vi "Serial Write and Read.vi"() -> ()   [LabVIEW 2019]
doc: "This example performs writes and reads on a serial port, as directed by the user. You can press the Write and Read buttons, and change the Read Count, while the example is running.\n\nThe parameters set for the serial port must match the parameters of the connected instrument or device. In this example, the Read Count parameter specifies the number of bytes that the serial port reads. If there were more bytes at the port than the specified number, those bytes would not be read. If there were less bytes at the port than the specified number, you would receive a timeout error.\n\nThis example expands upon the flow control options for XON and XOFF, allowing the user to choose those control characters. Also, the user can enable or disable a termination character. Some devices require a termination character in order to identify the end of command strings. Some devices send a termination character to signify the end of data to be read. This example shows how you can end the Read operation once a termination character is detected in the buffer and/or append a termination character at the end of the Write data."
uses:
  C:/Program Files (x86)/National Instruments/LabVIEW 2019/examples/Instrument IO/Serial/support/Serial - Settings.ctl
  <vilib>/Math Plots/3D Math Plots/3D Surface/3D Surface XCtrl/3D Surface.xctl
  <vilib>/Instr/_visa.llb/VISA Configure Serial Port (Instr).vi
  <vilib>/Math Plots/3D Math Plots/3D Surface/3D Surface Datatype/Public/Plot Helper (Vector).vi
  <vilib>/Utility/file.llb/Write Delimited Spreadsheet (string).vi
  <vilib>/Analysis/NI_AALBase.lvlib
  <vilib>/Math Plots/3D Math Plots/3D Surface/3D Surface Datatype/3D Surface Datatype.lvclass
panel:
  out "Noisy Pixel List":i32[][](array[numeric])
  out "Elapsed Time":dbl format="%#_g s"
  out "Intensity Graph":u32[][](graph)
  out "Cleaned Data":string[](array[string])
  out "Numeric Control":i32
  out "3D Surface":refnum<class "3D Plot Datatype.lvclass">[](xcontrol)
  out "output array":u32[][](array[numeric])
  out "appended array":u32[][](array[numeric])
  out "Histogram Graph":T1(graph)
  out "Channel":u32[](array[numeric])
  out "Energy":u32[](array[numeric])
  out "Chan+Energy":u32[](array[numeric]) format="%.0x"
  out "Clk Ticks":u32[](array[numeric])
  out "Sr No":u32[](array[numeric])
  out "Data+Garbage":string[](array[string])
  in  "Write":bool
  in  "Command":string="¡ÿU"
  in  "Read Termination Character":u8=10 format="%.0x"
  in  "Stop":bool
  in  "Read Count":u32=1000
  out "Response":string
  in  "Read":bool
  in  "Serial Settings":T2={"baud rate"=115200, "data bits"=8, "parity"=enum."None", "stop bits"=10, "flow control"=0} {"flow control" items=["None"=0, "XON/XOFF"=1, "RTS/CTS"=2, "DTR/DSR"=4]; "stop bits" items=["1.0"=10, "1.5"=15, "2.0"=20]; "data bits" min=5 max=8 step=1; "baud rate" items=["75"=75, "110"=110, "134"=134, "150"=150, "300"=300, "600"=600, "1200"=1200, "1800"=1800, "2400"=2400, "4800"=4800, "7200"=7200, "9600"=9600, "14400"=14400, "19200"=19200, "28800"=28800, "38400"=38400, "56000"=56000, "57600"=57600, "115200"=115200, "128000"=128000, "230400"=230400]}
  in  "End Read on Termination Character?":bool=TRUE
  in  "VISA resource name":refnum<visa-resource-name>="COM6"
  # "Overview: Demonstrates the use of the VISA functions to write commands to and read responses from a serial instrument continuously in a loop.\nRequirements: NI-VISA Driver\nInstructions:\n1. Run the VI.\n2. Specify a Command and click the Write button.\n3. Read a Response by clicking the Read button.\n4. Click Stop to stop the VI."
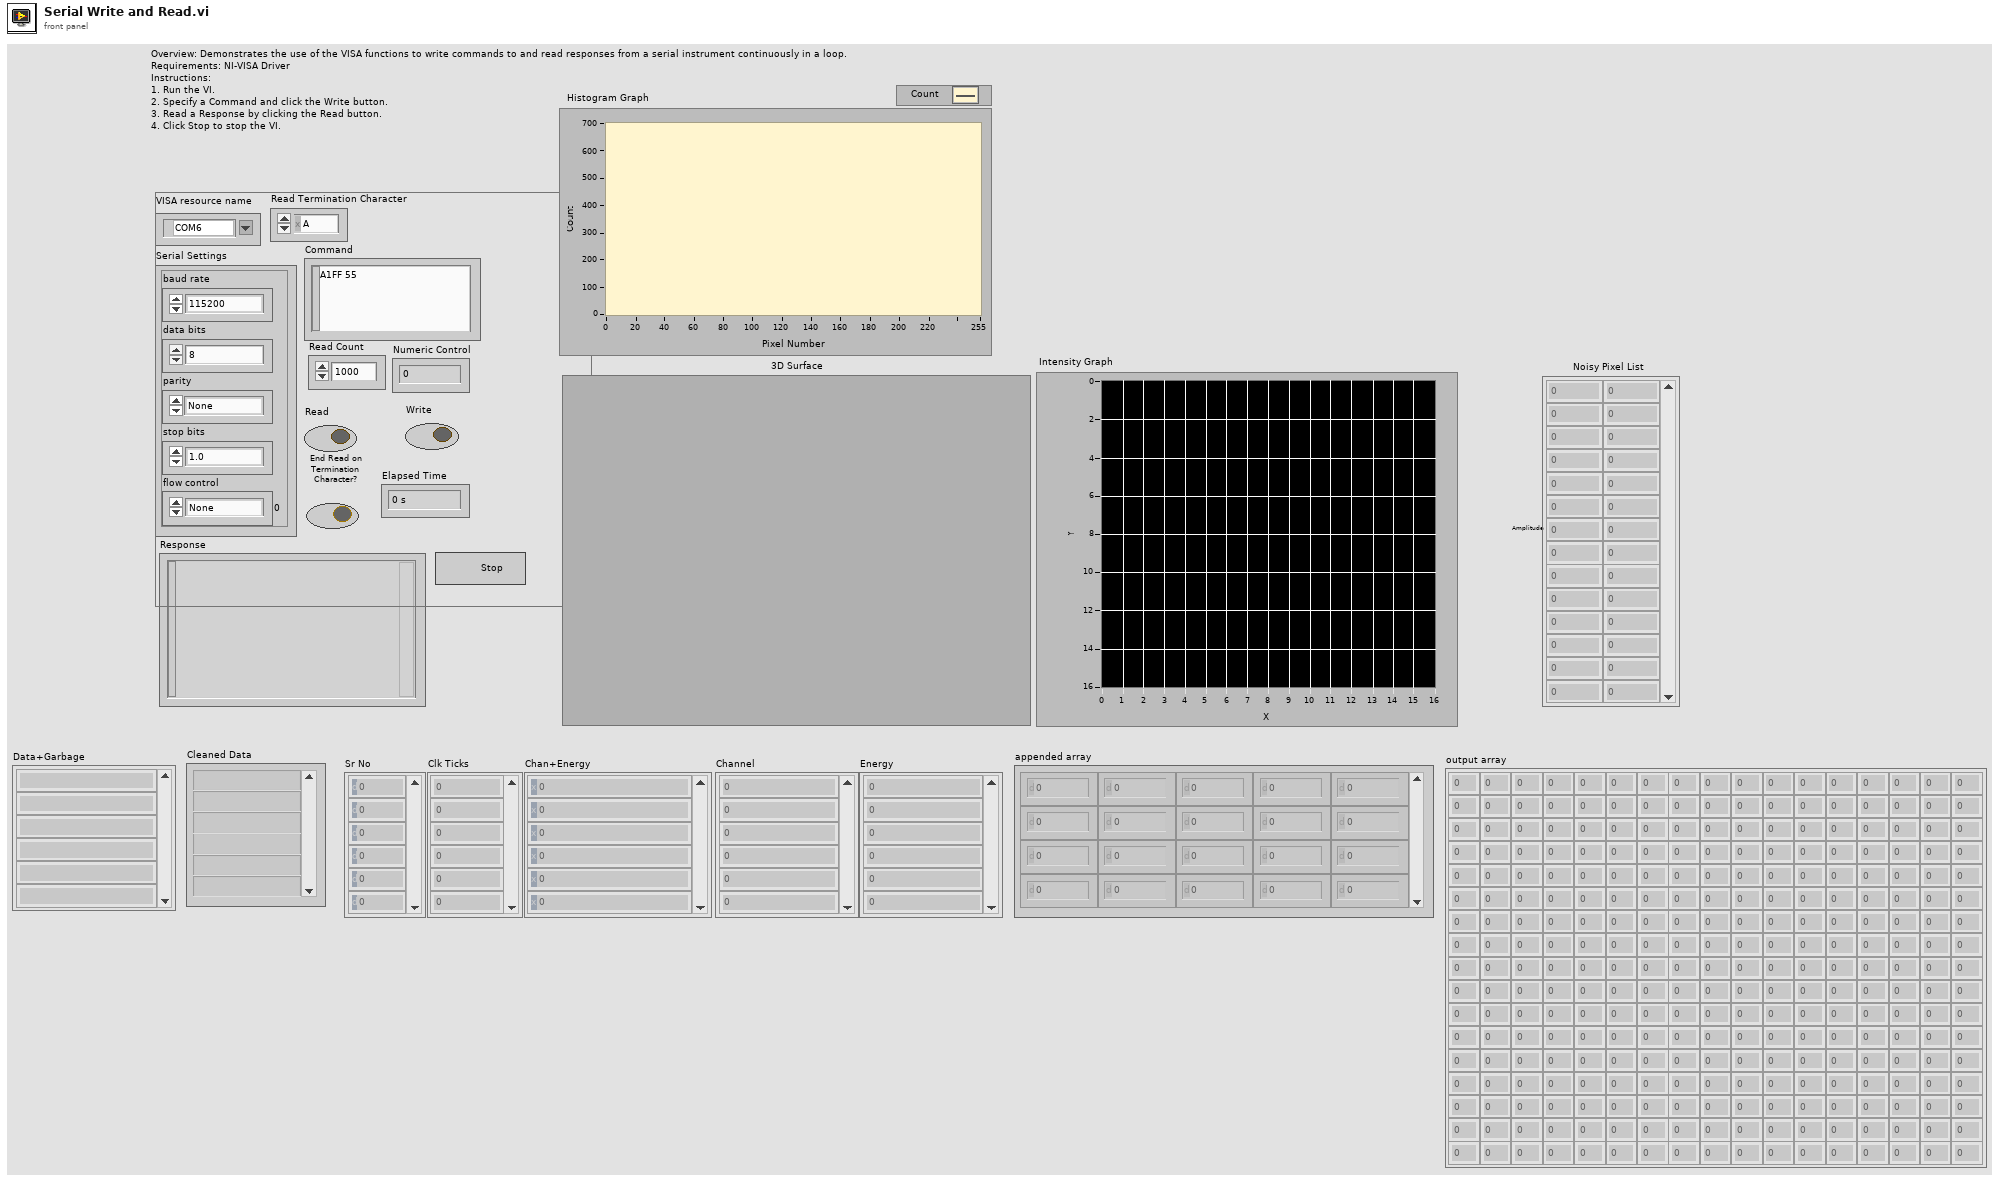
[diagram p1: front panel]
types:
  T1 = cluster{"X Values":dbl[], "Histogram: h(x)":i32[]}
  T2 = typedef "Serial - Settings.ctl" = cluster{"baud rate":u32, "data bits":u16, "parity":enum16{"None", "Odd", "Even", "Mark", "Space"}, "stop bits":u16, "flow control":u16}
  T3 = enum16{"open", "replace", "create", "open or create", "replace or create", "replace or create with confirmation"}
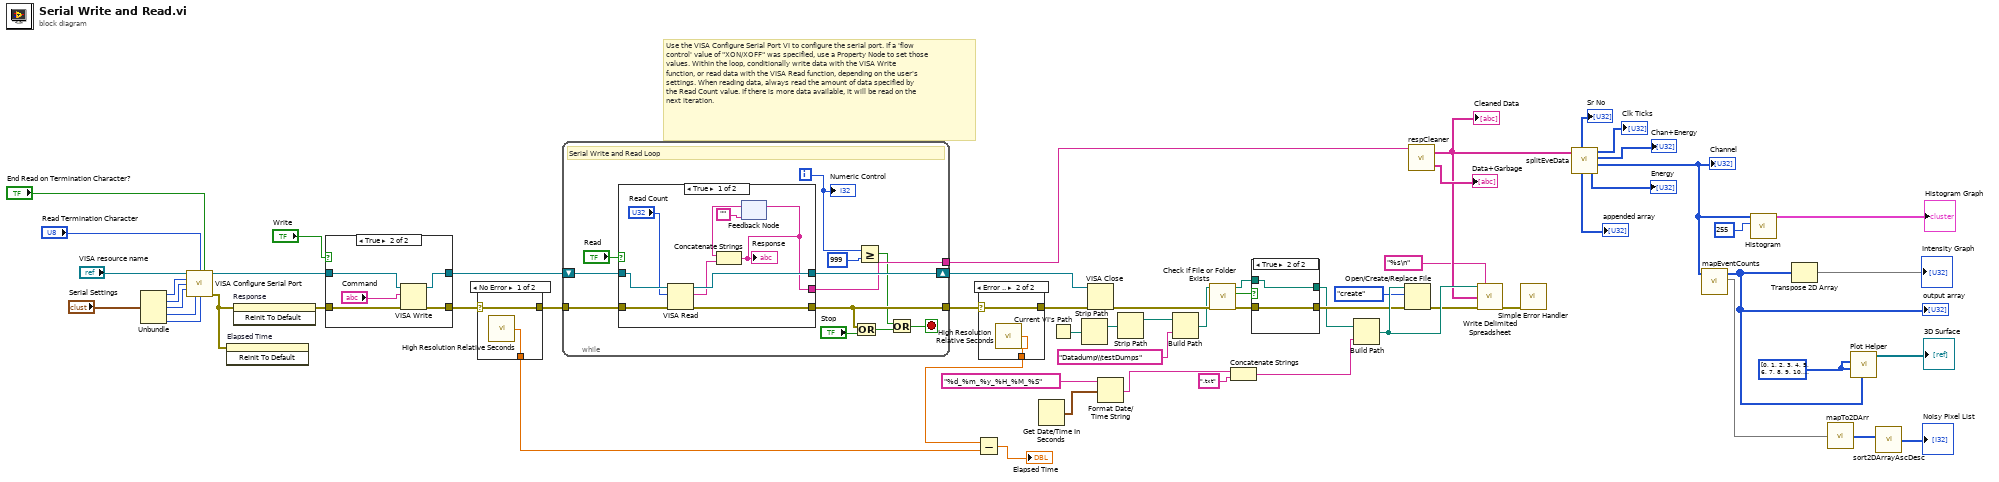
[diagram p0: block diagram]
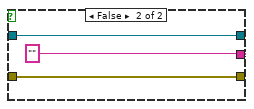
[diagram p2: hidden frame]
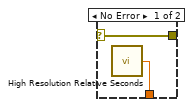
[diagram p5: hidden frame]
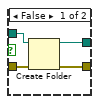
[diagram p6: hidden frame]
diagram:
  w47 = u8[] [0, 1, 2, 3, 4, 5, 6, 7, 8, 9, 10, 11, 12, 13, 14, 15, 0, 1, 2, 3, 4, 5, 6, 7, 8, 9, 10, 11, 12, 13, 14, 15, 0, 1, 2, 3, 4, 5, 6, 7, 8, 9, 10, 11, 12, 13, 14, 15, 0, 1, 2, 3, 4, 5, 6, 7, 8, 9, 10, 11, 12, 13, 14, 15, 0, 1, 2, 3, 4, 5, 6, 7, 8, 9, 10, 11, 12, 13, 14, 15, 0, 1, 2, 3, 4, 5, 6, 7, 8, 9, 10, 11, 12, 13, 14, 15, 0, 1, 2, 3, 4, 5, 6, 7, 8, 9, 10, 11, 12, 13, 14, 15, 0, 1, 2, 3, 4, 5, 6, 7, 8, 9, 10, 11, 12, 13, 14, 15, 0, 1, 2, 3, 4, 5, 6, 7, 8, 9, 10, 11, 12, 13, 14, 15, 0, 1, 2, 3, 4, 5, 6, 7, 8, 9, 10, 11, 12, 13, 14, 15, 0, 1, 2, 3, 4, 5, 6, 7, 8, 9, 10, 11, 12, 13, 14, 15, 0, 1, 2, 3, 4, 5, 6, 7, 8, 9, 10, 11, 12, 13, 14, 15, 0, 1, 2, 3, 4, 5, 6, 7, 8, 9, 10, 11, 12, 13, 14, 15, 0, 1, 2, 3, 4, 5, 6, 7, 8, 9, 10, 11, 12, 13, 14, 15, 0, 1, 2, 3, 4, 5, 6, 7, 8, 9, 10, 11, 12, 13, 14, 15, 0, 1, 2, 3, 4, 5, 6, 7, 8, 9, 10, 11, 12, 13, 14] ("Array")
  # "Use the VISA Configure Serial Port VI to configure the serial port. If a 'flow control' value of \"XON/XOFF\" was specified, use a Property Node to set those values. Within the loop, conditionally write data with the VISA Write function, or read data with the VISA Read function, depending on the user's settings. When reading data, always read the amount of data specified by the Read Count value. If there is more data available, it will be read on the next iteration."
  n1 = Unbundle("Serial Settings") -> ("baud rate"=w57:u32, "data bits"=w58:u16, "parity"=w59:enum16{"None", "Odd", "Even", "Mark", "Space"}, "stop bits"=w60:u16, "flow control"=w53:u16)
  n2 = call-poly "VISA Configure Serial Port"("VISA resource name"="VISA resource name", "termination char\n(0xA = '\\n' = LF)"="Read Termination Character", "Enable Termination\nChar (T)"="End Read on Termination Character?", "baud rate (9600)"=w57, "data bits (8)"=w58, "parity (0:none)"=w59, "stop bits (10: 1 bit)"=w60, "flow control (0:none)"=w53) -> ("VISA resource name out"=w52:refnum<visa-resource-name>, "error out"=w15:errorcluster)  [unwired: 2 in, 4 out]
  n3 = invoke on="Elapsed Time" class="DigNum (strict)" method="Reinit To Default"(error in=w15) -> ()  [unwired: 2 in, 3 out]
  n4 = invoke on="Response" class="Str" method="Reinit To Default"(error in=w15) -> (error out=w49:errorcluster)  [unwired: 2 in, 2 out]
  n5 = case shown="True" "Write" {
    tunnel: w52 -> [w63 w67]
    tunnel: w49 -> [w62 w66]
    tunnel: [w63 w65] -> w7
    tunnel: [w62 w64] -> w6
    frame False {
    }
    frame True {
      n6 = VISA Write(VISA resource name=w67, write buffer="Command", error in (no error)=w66) -> (VISA resource name out=w65:refnum<visa-resource-name>, error out=w64:errorcluster)  [unwired: 1 out]
    }
  }
  n7 = case shown="No Error" w6 {
    selector: w6 -> [w70 w71]
    tunnel: [w70 w71] -> w5
    tunnel: [w69 _] -> w19
    frame No Error {
      n8 = call <vilib>:"High Resolution Relative Seconds.vi"() -> ("relative seconds"=w69:dbl)
    }
    frame Error {
    }
  }
  n9 = while {
    shift-right: [w83] -> w54
    shift-left: w7 -> [w79]
    tunnel: w5 -> [w78]
    tunnel: [w81] -> w20
    tunnel: [w77] -> w32
    i -> [w76]
    stop <- w72 stop-if-true
    # "Serial Write and Read Loop"
    n10 = case shown="True" "Read" {
      tunnel: [w90 w95] -> w83
      tunnel: w79 -> [w92 w95]
      tunnel: [w88 w94] -> w81
      tunnel: w78 -> [w91 w94]
      tunnel: [w84 ""] -> w77
      frame True {
        n11 = VISA Read(VISA resource name=w92, byte count="Read Count", error in (no error)=w91) -> (VISA resource name out=w90:refnum<visa-resource-name>, read buffer=w87:string, error out=w88:errorcluster)  [unwired: 1 out]
        n12 = feedback #1("") -> (w86:string)
        n13 = Concatenate Strings(w86, w87) -> (w84:string)
        "Response" <- w84
        n14 = feedback-in #1(w84) -> ()
      }
      frame False {
      }
    }
    n15 = Or(x=w81, y="Stop") -> (x .or. y?=w73:bool)
    n16 = Greater Or Equal?(x=w76, y=999) -> (x >= y?=w74:bool)
    n17 = Or(x=w74, y=w73) -> (x .or. y?=w72:bool)
    "Numeric Control" <- w76
  }
  n18 = case shown="Error .." w20 {
    selector: w20 -> [w97 w99]
    tunnel: [w97 w99] -> w21
    tunnel: [w96 w98] -> w18
    frame No Error {
      n19 = call <vilib>:"High Resolution Relative Seconds.vi"() -> ("relative seconds"=w96:dbl)
    }
    frame Error {
      n20 = call <vilib>:"High Resolution Relative Seconds.vi"() -> ("relative seconds"=w98:dbl)
    }
  }
  n21 = Subtract(x=w18, y=w19) -> (x-y=→"Elapsed Time":dbl)
  n22 = Get Date/Time In Seconds() -> (seconds since 1Jan1904=w42:timestamp)
  n23 = Current VI's Path() -> (path=w44:path)
  n24 = Strip Path(path=w44) -> (stripped path=w34:path)  [unwired: 1 out]
  n25 = VISA Close(VISA resource name=w54, error in (no error)=w21) -> (error out=w14:errorcluster)
  n26 = Format Date/Time String(time format string (%c)="%d_%m_%y_%H_%M_%S", seconds (now)=w42) -> (date/time string=w40:string)  [unwired: 1 in]
  n27 = Strip Path(path=w34) -> (stripped path=w33:path)  [unwired: 1 out]
  n28 = Build Path(base path=w33, name or relative path="Datadump\\testDumps") -> (appended path=w13:path)
  n29 = call <vilib>:"Check if File or Folder Exists.vi"("error in (no error)"=w14, "path"=w13) -> ("error out"=w12:errorcluster, "file or folder exists?"=w9:bool, "dup path"=w10:path)  [unwired: 7 in]
  n30 = Concatenate Strings(w40, ".txt") -> (w38:string)
  n31 = case shown="True" w9 {
    tunnel: w12 -> [w103 w105]
    tunnel: w10 -> [w102 w104]
    tunnel: [w101 w105] -> w11
    tunnel: [w100 w104] -> w8
    frame False {
      n32 = Create Folder(path (use dialog)=w102, error in=w103) -> (created path=w100:path, error out=w101:errorcluster)  [unwired: 1 in, 1 out]
    }
    frame True {
    }
  }
  n33 = Build Path(base path=w8, name or relative path=w38) -> (appended path=w37:path)
  n34 = Open/Create/Replace File(file path (use dialog)=w37, error in=w11, operation (0:open)=T3."create") -> (error out=w36:errorcluster)  [unwired: 3 in, 2 out]
  n35 = call "respCleaner.vi"("Raw Response"=w32) -> ("Data+Garbage"=→"Data+Garbage":string[], "Clean Data"=w23:string[])  [unwired: 3 in]
  "Cleaned Data" <- w23
  n36 = call-poly <vilib>:"Write Delimited Spreadsheet.vi"("file path (dialog if empty)"=w37, "format (%s)"="%s\n", "1D data"=w23, "error in (no error)"=w36) -> ("error out"=w45:errorcluster)  [unwired: 10 in, 1 out]
  n37 = call <vilib>:"Simple Error Handler.vi"("error in (no error)"=w45) -> ()  [unwired: 1 in, 8 out]
  n38 = call "splitEveData.vi"("Clean Data Array"=w23) -> ("Energy"=→"Energy":u32[], "Channel"=w24:u32[], "Chan+Energy"=→"Chan+Energy":u32[], "Clk Ticks"=→"Clk Ticks":u32[], "appended array"=→"appended array":u32[][], "Sr No"=→"Sr No":u32[])  [unwired: 3 in]
  "Channel" <- w24
  n39 = call "mapEventCounts.vi"("Count"=w24) -> ("Counts (map)"=w3:map{u32, u32}, "Count Grid"=w4:u32[][])  [unwired: 3 in]
  "output array" <- w4
  n40 = call <vilib>:"Histogram.vi"("intervals"=255, "X"=w24) -> ("Histogram Graph"=→"Histogram Graph":T1)  [unwired: 5 in, 4 out]
  n41 = Transpose 2D Array(2D array=w4) -> (transposed array=→"Intensity Graph":u32[][])
  n42 = call "mapTo2DArr.vi"("Map"=w3) -> ("2D Array"=w1:i32[][])
  n43 = call-poly <vilib>:"Plot Helper.vi"("z matrix"=w4, "y vector"=w47, "x vector"=w47) -> ("3D Plot lvclass Array out"=→"3D Surface":refnum<class "3D Plot Datatype.lvclass">[])  [unwired: 3 in, 5 out]
  n44 = call "sort2DArrayAscDesc.vi"("2D Array"=w1) -> ("sorted 2D array"=→"Noisy Pixel List":i32[][])  [unwired: 5 in]
